vi "Get Attributes.vi"(8 "error in (no error)":errorcluster, 10 "Only Get DVR Reference":bool, 11 "reference in":refnum<class "Websocket.lvclass">) -> (0 "error out":errorcluster, 1 "DataRef":refnum<data-value>, 2 "Data":T1, 3 "reference out":refnum<class "Websocket.lvclass">)   [LabVIEW 2017, in "Front Panel Publisher.lvlib" / "Websocket.lvclass"]
uses:
  Websocket.lvclass
  Protected/Object Attributes.ctl
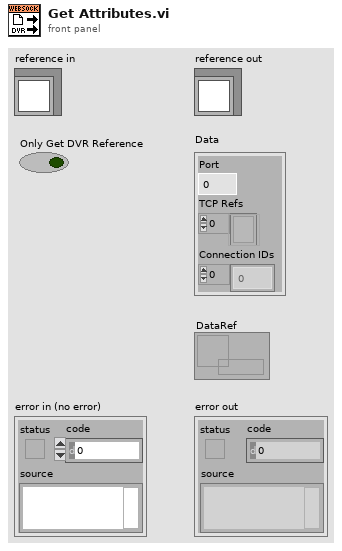
[diagram p1: front panel]
types:
  T1 = typedef "Front Panel Publisher.lvlib/Websocket.lvclass/Object Attributes.ctl" = cluster{"Port":u16, "TCP Refs":refnum<k5>[], "Connection IDs":u64[]}
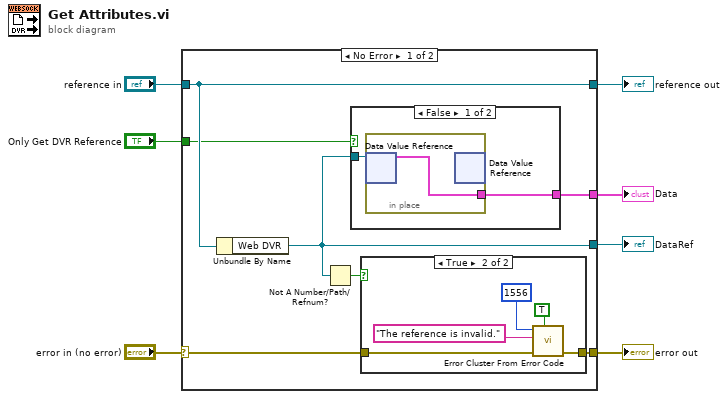
[diagram p0: block diagram]
diagram:
  n1 = case shown="No Error" "error in (no error)" {
    selector: "error in (no error)" -> [w11 w24]
    tunnel: [w10 w24] -> w6
    tunnel: [w14 w25] -> w4
    tunnel: "reference in" -> [w14 w25]
    tunnel: [w9 _] -> w3
    tunnel: "Only Get DVR Reference" -> [w13 _]
    tunnel: [w8 _] -> w1
    frame No Error {
      n2 = Unbundle By Name(w14) -> ("Web DVR"=w9:refnum<data-value>)
      n3 = Not A Number/Path/Refnum?(number/path/refnum=w9) -> (NaN/Path/Refnum?=w12:bool)
      n4 = case shown="False" w13 {
        tunnel: w9 -> [w22 _]
        tunnel: [w21 _] -> w8
        frame False {
          n5 = in-place {
            in-place-border: [w23] -> w21
            n6 = in-place-dvr #1(w22) -> (w23:T1)  [unwired: 1 out]
            n7 = in-place-dvr #1() -> ()  [unwired: 1 in, 2 out]
          }
        }
        frame True {
        }
      }
      n8 = case shown="True" w12 {
        tunnel: w11 -> [w15 w17]
        tunnel: [w15 w16] -> w10
        frame False {
        }
        frame True {
          n9 = call <vilib>:"Error Cluster From Error Code.vi"("show call chain? (False)"=TRUE, "error in (no error)"=w17, "error message (\"\")"="The reference is invalid." ("source"), "error code (0)"=1556 ("code")) -> ("error out"=w16:errorcluster)  [unwired: 5 in]
        }
      }
    }
    frame Error {
    }
  }
  "error out" <- w6
  "reference out" <- w4
  "DataRef" <- w3
  "Data" <- w1
